vi "Configure Acquisition Type Core.vi"(8 "error in (no error)":errorcluster, 10 "acquisition type (Normal)":i32(ring) items=["Normal", "Peak Detect", "High Resolution", "Envelope", "Average"], 11 "CS++Scope":refnum<class "CS++Scope.lvclass">) -> (0 "error out":errorcluster, 3 "CS++Scope out":refnum<class "CS++Scope.lvclass">)   [LabVIEW 2015, in "CS++Scope.lvlib" / "CS++Scope.lvclass"]
doc: "This VI configures how the oscilloscope acquires data and how it fills the waveform record."
uses:
  CS++Scope.lvclass
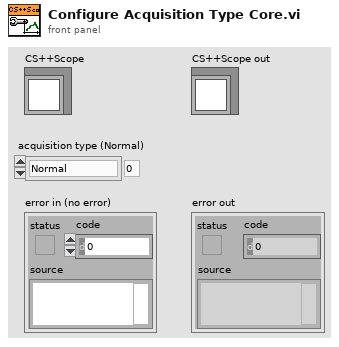
[diagram p1: front panel]
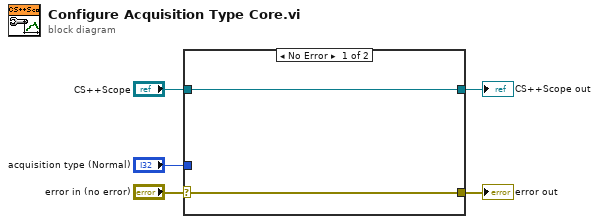
[diagram p0: block diagram]
diagram:
  n1 = case shown="No Error" "error in (no error)" {
    selector: "error in (no error)" -> [w6 w9]
    tunnel: [w6 w9] -> w4
    tunnel: [w7 w8] -> w2
    tunnel: "CS++Scope" -> [w7 w8]
    tunnel: "acquisition type (Normal)" -> [_ _]
    frame No Error {
    }
    frame Error {
    }
  }
  "error out" <- w4
  "CS++Scope out" <- w2
